vi "init.vi"(8 "error in (no error)":errorcluster, 9 "ID Query (True)":bool=TRUE, 10 "Serial Configuration":T1={"Baud Rate"=115200, "Flow Control"=0, "Parity"=0, "Stop Bits"=10, "Data Bits"=8} {"Stop Bits" items=["1.0"=10, "1.5"=15, "2.0"=20]; "Parity" items=["None", "Odd", "Even", "Mark", "Space"]; "Flow Control" items=["None", "XON/XOFF", "RTS/CTS"]}, 11 "VISA resource name":refnum<visa-resource-name>) -> (0 "error out":errorcluster, 1 "IDN result":string, 3 "VISA resource name out":refnum<visa-resource-name>)   [LabVIEW 2023]
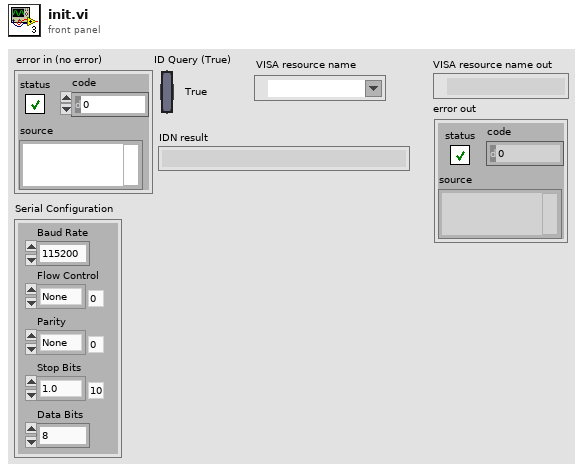
[diagram p1: front panel]
types:
  T1 = cluster{"Baud Rate":u32, "Flow Control":u16, "Parity":u16, "Stop Bits":u16, "Data Bits":u16}
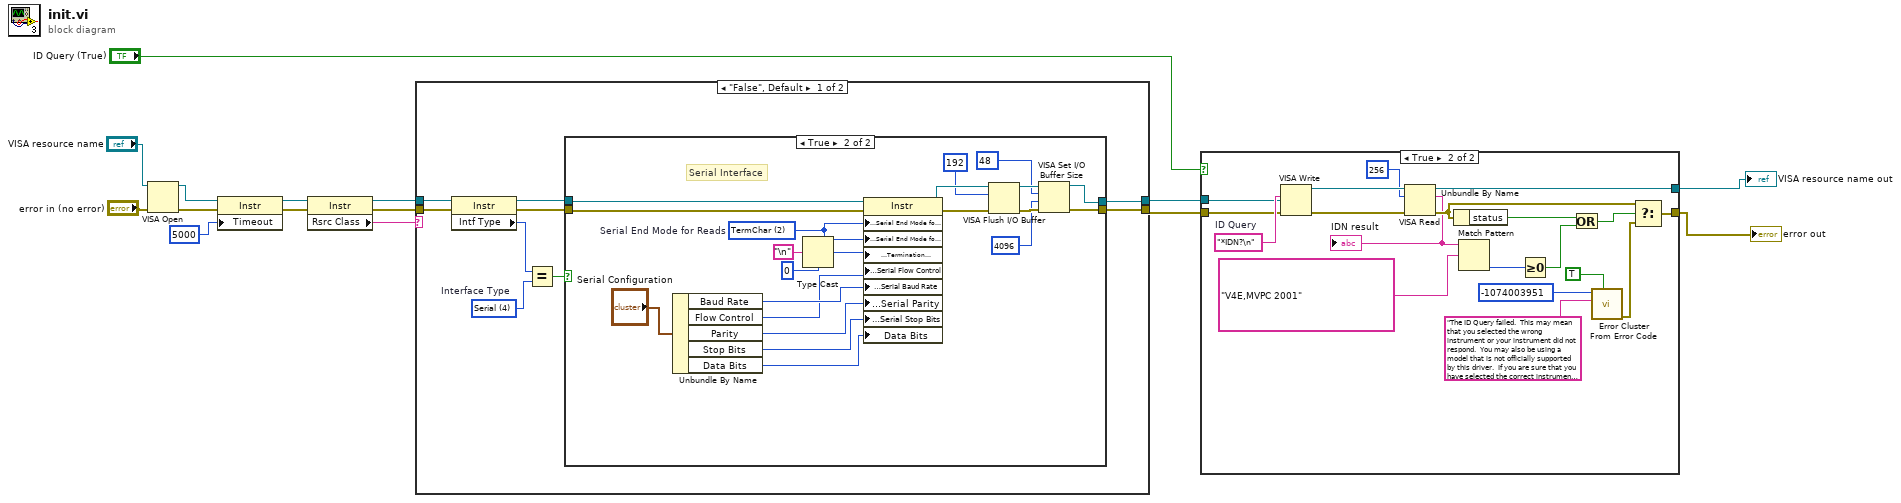
[diagram p0: block diagram]
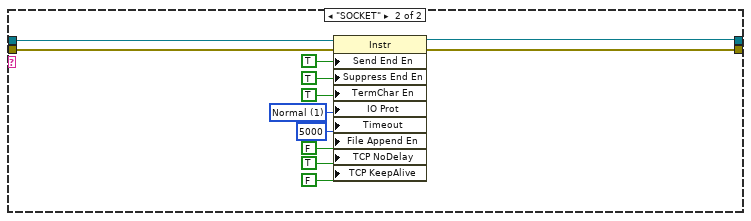
[diagram p3: hidden frame]
diagram:
  n1 = VISA Open(error in (no error)="error in (no error)", VISA resource name="VISA resource name") -> (VISA resource name=w6:refnum<visa-resource-name>, error out=w5:errorcluster)  [unwired: 3 in]
  n2 = property class="Instr"(reference=w6, error in=w5, "Timeout"=u32 5000 ("General Settings:Timeout Value")) -> (reference out=w3:refnum<visa-resource-name>, error out=w4:errorcluster)
  n3 = property class="Instr"(reference=w3, error in=w4) -> (reference out=w11:refnum<visa-resource-name>, error out=w10:errorcluster, "Rsrc Class"=w12:string)
  n4 = case shown="\"False\", Default" w12 {
    tunnel: w11 -> [w24 w56]
    tunnel: w10 -> [w23 w55]
    tunnel: [w21 w58] -> w9
    tunnel: [w20 w57] -> w8
    frame "False", Default {
      w18 = u16 4 items=["GPIB"=1, "VXI"=2, "GPIB-VXI"=3, "Serial"=4, "PXI"=5, "TCPIP"=6, "USB"=7, "FireWire"=9]  # Interface Type
      n5 = property class="Instr"(reference=w24, error in=w23) -> (reference out=w17:refnum<visa-resource-name>, error out=w22:errorcluster, "Intf Type"=w19:u16)
      n6 = Equal?(x=w19, y=w18) -> (x = y?=w16:bool)
      n7 = case shown="True" w16 {
        tunnel: w22 -> [w26 w36]
        tunnel: [w25 w35] -> w21
        tunnel: [w26 w34] -> w20
        tunnel: w17 -> [w25 w33]
        frame False {
        }
        frame True {
          w38 = u16 2 items=["None", "LastBit", "TermChar"]  # Serial End Mode for Reads
          # "Serial Interface"
          n8 = Unbundle By Name("Serial Configuration") -> ("Baud Rate"=w31:u32, "Flow Control"=w30:u16, "Parity"=w29:u16, "Stop Bits"=w28:u16, "Data Bits"=w27:u16)
          n9 = Type Cast(type=u8 0, x="\n") -> (*(type *) &x=w37:u8)
          n10 = property class="Instr"(reference=w33, error in=w36, "Serial Settings:Serial End Mode for Reads"=w38, "Serial Settings:Serial End Mode for Writes"=w38, "Message Based Settings:Termination Character"=w37, "Serial Settings:Serial Flow Control"=w30, "Serial Settings:Serial Baud Rate"=w31, "Serial Settings:Serial Parity"=w29, "Serial Settings:Serial Stop Bits"=w28, "Data Bits"=w27) -> (reference out=w44:refnum<visa-resource-name>, error out=w46:errorcluster)
          n11 = VISA Flush I/O Buffer(VISA resource name=w44, mask (16)=u16 192, error in (no error)=w46) -> (VISA resource name out=w47:refnum<visa-resource-name>, error out=w45:errorcluster)
          n12 = VISA Set I/O Buffer Size(VISA resource name=w47, mask (16)=u16 48, size (4096)=u32 4096 ("size (0)"), error in (no error)=w45) -> (VISA resource name out=w35:refnum<visa-resource-name>, error out=w34:errorcluster)
        }
      }
    }
    frame "SOCKET" {
      w51 = u16 1 items=["Normal"=1, "VXI/FDC"=2, "GPIB/HS488"=3, "Serial-TCPIP-USB/488 Strings"=4, "USBTMC/Vendor-Specific"=5] ("Message Based Settings:IO Protocol")
      n13 = property class="Instr"(reference=w56, error in=w55, "Send End En"=TRUE ("Message Based Settings:Termination Character Enable"), "Suppress End En"=TRUE ("Message Based Settings:Suppress End Enable"), "TermChar En"=TRUE ("Message Based Settings:Termination Character Enable"), "IO Prot"=w51, "Timeout"=u32 5000 ("General Settings:Timeout Value"), "File Append En"=FALSE ("Message Based Settings:File Append Enable"), "TCP NoDelay"=TRUE ("TCP/IP Settings:No Packet Delay"), "TCP KeepAlive"=FALSE ("TCP/IP Settings:Keep-Alive Packets")) -> (reference out=w58:refnum<visa-resource-name>, error out=w57:errorcluster)
    }
  }
  n14 = case shown="True" "ID Query (True)" {
    tunnel: [w60 w80] -> w1
    tunnel: [w61 w79] -> w2
    tunnel: w9 -> [w61 w64]
    tunnel: w8 -> [w60 w63]
    frame False {
    }
    frame True {
      w74 = "*IDN?\n"  # ID Query
      n15 = VISA Write(VISA resource name=w64, write buffer=w74, error in (no error)=w63) -> (VISA resource name out=w78:refnum<visa-resource-name>, error out=w77:errorcluster)  [unwired: 1 out]
      n16 = VISA Read(VISA resource name=w78, byte count=u32 256, error in (no error)=w77) -> (VISA resource name out=w79:refnum<visa-resource-name>, read buffer=w62:string, error out=w68:errorcluster)  [unwired: 1 out]
      "IDN result" <- w62
      n17 = Unbundle By Name(w68) -> ("status"=w67:bool)
      n18 = Match Pattern(string=w62, regular expression="V4E,MVPC 2001") -> (offset past match=w69:i32)  [unwired: 1 in, 3 out]
      n19 = Greater Or Equal To 0?(x=w69) -> (x >= 0?=w66:bool)
      n20 = Or(x=w67, y=w66) -> (x .or. y?=w65:bool)
      n21 = call <vilib>:"Error Cluster From Error Code.vi"("show call chain? (False)"=TRUE, "error message (\"\")"="The ID Query failed.  This may mean that you selected the wrong instrument or your instrument did not respond.  You may also be using a model that is not officially supported by this driver.  If you are sure that you have selected the correct instrument and it is responding, try disabling the ID Query." ("Source (VI Name)"), "error code (0)"=-1074003951 ("Code")) -> ("error out"=w73:errorcluster)  [unwired: 6 in]
      n22 = Select(t=w68, s=w65, f=w73) -> (s? t:f=w80:errorcluster)
    }
  }
  "VISA resource name out" <- w2
  "error out" <- w1
